vi "Wavelet Packet - Plot Tree.vi"() -> ()   [LabVIEW 2023]
doc: "This example shows how to plot a wavelet packet tree by using the WA WP Plot Tree VI. \n\n<b>Instructions:</b>\n1) Run this VI.\n2) Change the value of <b>Level</b> to plot a wavelet packet decomposition tree at different levels. \n3) Change the <b>Display Mode</b> to select a different node label."
uses:
  <vilib>/addons/Wavelet Analysis/typedefs.llb/WA Data.ctl
  <vilib>/addons/Wavelet Analysis/wavelet packet.llb/WA WP Decomposition (Waveform).vi
  <vilib>/addons/_Advanced Signal Processing/NI_AdvSigProcWA.lvlib
panel:
  in  "stop":bool
  in  "Display Mode":u16(ring) items=["Node path", "Depth, position", "Entropy"]
  out "Wavelet Packet Tree":picture
  in  "Wavelet":u16(ring) items=["db02"=0, "db03"=1, "db04"=2, "db05"=3, "db06"=4, "db07"=5, "db08"=6, "db09"=7, "db10"=8, "db11"=9, "db12"=10, "db13"=11, "db14"=12, "Haar"=13, "bior1_3"=14, "bior1_5"=15, "bior2_2"=16, "bior2_4"=17, "bior2_6"=18, "bior2_8"=19, "bior3_1"=20, "bior3_3"=21, "bior3_5"=22, "bior3_7"=23, "bior3_9"=24, "bior4_4 (FBI)"=25, "bior5_5"=38, "bior6_8"=39, "coif1"=26, "coif2"=27, "coif3"=28, "coif4"=29, "coif5"=30, "sym2"=31, "sym3"=32, "sym4"=33, "sym5"=34, "sym6"=35, "sym7"=36, "sym8"=37]
  in  "Level":i32=3
  # "Overview: Shows how to plot a wavelet packet tree by using the WA WP Plot Tree VI.\nRequirements: LabVIEW Full Development System, Advanced Signal Processing Toolkit\nInstructions: \n1. Run this VI.\n2. Change the value of Level to plot a wavelet packet decomposition tree at different levels. \n3. Change the Display Mode to select a different node label.\n4. Click Stop to stop the VI."
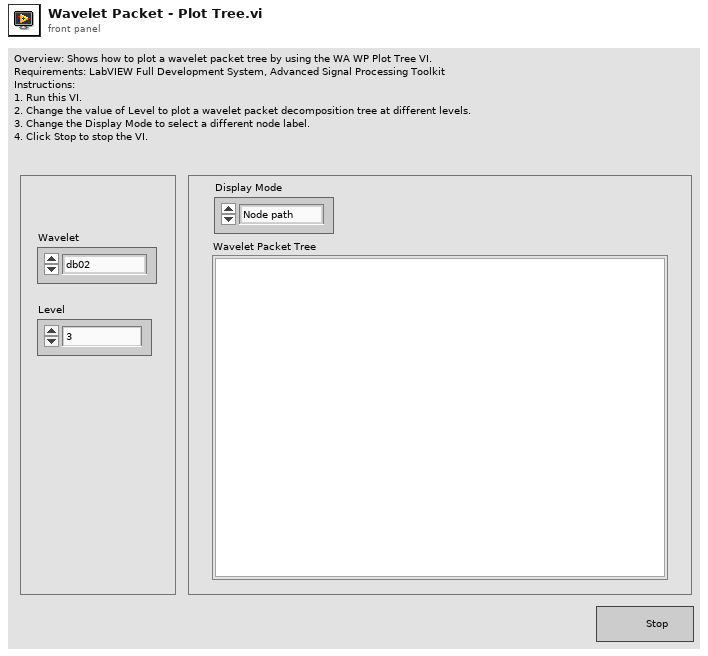
[diagram p1: front panel]
types:
  T1 = typedef "NI_AdvSigProcWA.lvlib/WA Generic Ref.ctl" = cluster{"ref":u64, "t0":timestamp, "dt":dbl}
  T2 = typedef "NI_AdvSigProcWA.lvlib/WA Data.ctl" = u16
  T3 = typedef "LVBoundsTypeDef.ctl" = cluster{"Width":u32, "Height":u32}
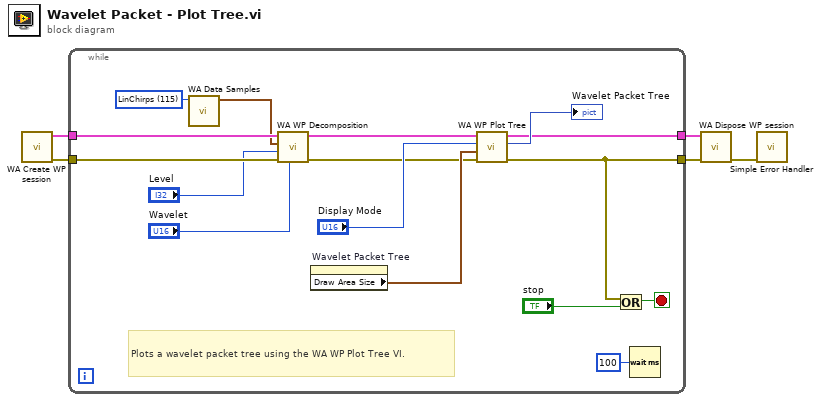
[diagram p0: block diagram]
diagram:
  n1 = call <vilib>:"WA Create WP session.vi"() -> ("error out"=w4:errorcluster, "WP session out"=w5:T1)  [unwired: 1 in, 9 out]
  n2 = while {
    tunnel: w5 -> [w21]
    tunnel: w4 -> [w20]
    tunnel: [w11] -> w3
    tunnel: [w7] -> w2
    stop <- w12 stop-if-true
    w8 = T2 115 items=["1D Example Data"=100, "-"=101, "Doppler"=102, "HOP"=103, "TF Sine"=104, "Noisy Doppler"=105, "Sea Temperature"=106, "Sp500"=107, "Power Line"=108, "Engine Knocking"=109, "HeaviSine"=110, "Bumps"=111, "Blocks"=112, "Piece Regular"=113, "HypChirps"=114, "LinChirps"=115, "Chirps"=116, "Piece Polynomial"=117, "ECG"=131, "-"=118, "2D Example Data"=119, "-"=120, "Finger Print (Image)"=121, "Iris Flower (Image)"=122, "Mammogram (Image)"=123, "Lake (Image)"=127, "Two Can 1 (Image)"=132, "Two Can 2 (Image)"=133, "Camera Man (Image)"=134] ("data")
    # "Plots a wavelet packet tree using the WA WP Plot Tree VI."
    n3 = call <vilib>:"WA Data Samples.vi"("data"=w8) -> ("signal"=w19:waveform(dbl))  [unwired: 10 out]
    n4 = call-poly <vilib>:"WA WP Decomposition.vi"("wavelet"="Wavelet", "error in (no error)"=w20, "levels"="Level", "signal"=w19, "WP session"=w21) -> ("error out"=w9:errorcluster, "WP session out"=w10:T1)  [unwired: 5 out]
    n5 = property on="Wavelet Packet Tree" class="Pict"() -> ("Draw Area Size"=w15:T3)  [unwired: 2 in, 2 out]
    n6 = call <vilib>:"WA WP Plot Tree.vi"("error in (no error)"=w9, "draw area size"=w15, "display mode"="Display Mode", "WP session"=w10) -> ("error out"=w7:errorcluster, "tree plot"=→"Wavelet Packet Tree":picture, "WP session out"=w11:T1)  [unwired: 5 out]
    n7 = Or(x=w7, y="stop") -> (x .or. y?=w12:bool)
    n8 = Wait (ms)(milliseconds to wait=u32 100) -> ()  [unwired: 1 out]
  }
  n9 = call <vilib>:"WA Dispose WP session.vi"("error in (no error)"=w2, "WP session"=w3) -> ("error out"=w1:errorcluster)  [unwired: 9 out]
  n10 = call <vilib>:"Simple Error Handler.vi"("error in (no error)"=w1) -> ()  [unwired: 1 in, 8 out]
